vi "set_home_end.vi"(5 "End transform offset":dbl[](array[numeric])=[0.0, 0.0, 0.0, 0.0, 0.0, 0.0] format="%#.3f", 6 "End transform coordinates":T2(ring), 7 "Home pose offset":dbl[](array[numeric])=[0.0, 0.0, 0.0, 0.0, 0.0, 0.0] format="%#.3f", 9 "Probe pose (ASAP)":T1, 10 "Probe rotation (stage)":T1, 11 "Pivot point (mm)":dbl[](array[numeric])) -> (1 "End transform string":string, 2 "End transform":dbl[](array[numeric]), 3 "Home pose":dbl[](array[numeric]))   [LabVIEW 2013]
uses:
  <vilib>/Analysis/Matrix/Datatypes/RealMatrix.ctl
  <vilib>/Analysis/baseanly.llb/Real A x B.vi
  initialization/micron_globals.vi
  <vilib>/Analysis/NI_AALBase.lvlib
  <vilib>/Analysis/Matrix/NI_Matrix.lvlib
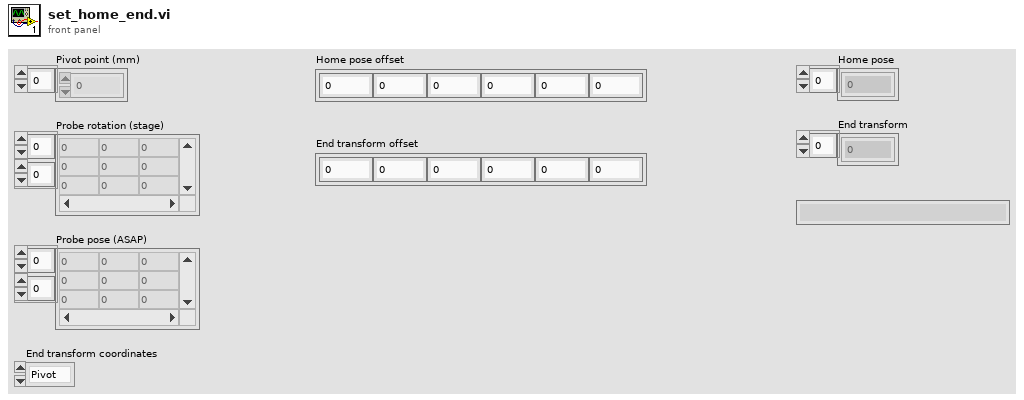
[diagram p1: front panel]
types:
  T1 = typedef "NI_Matrix.lvlib/RealMatrix.ctl" = dbl[][]
  T2 = enum16{"Pivot", "Probe", "ASAP", "Sensor 0", "Sensor 1"}
  T3 = typedef "configuration.ctl" = cluster{"Calibration data":T4, "Block size":i32, "Tasks":cluster{"Analog Input":refnum<k21>, "Counters":refnum<k21>[], "Digital out":refnum<k21>}, "Light enables":bool[]}
  T4 = typedef "asap_calibration.ctl" = cluster{"T1":T1, "K1":T1, "T2":T1, "K2":T1, "Sensor LUT":sgl[][][][]}
  T5 = typedef "motion_status.ctl" = cluster{"Axis names":string[], "Axis positions":dbl[], "Pose":dbl[], "Timestamp":u32, "Ready":bool, "Stopped":bool}
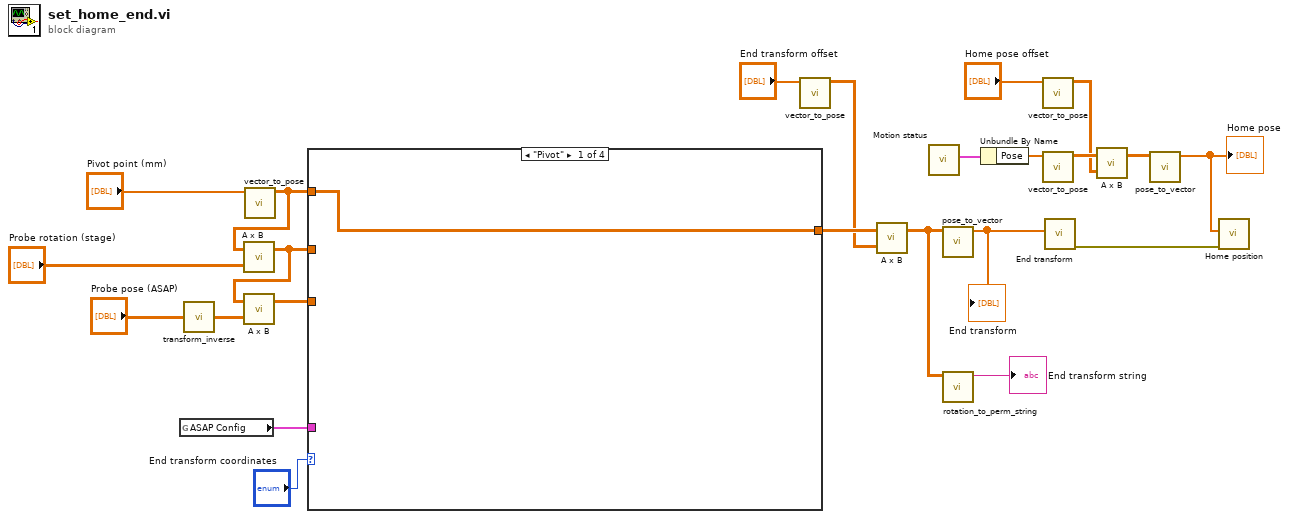
[diagram p0: block diagram]
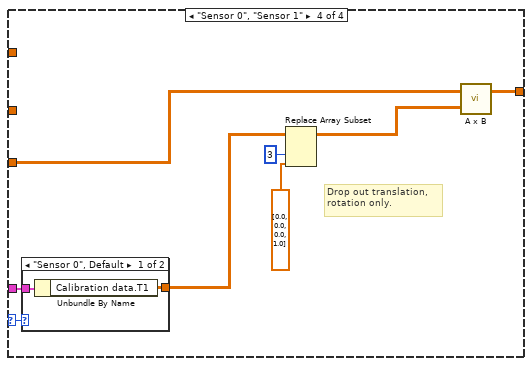
[diagram p4: hidden frame]
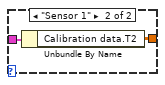
[diagram p5: hidden frame]
diagram:
  n1 = global read "micron_globals.vi" "ASAP Config"() -> (w13:T3)
  n2 = call "transform_inverse.vi"("Transform"="Probe pose (ASAP)") -> ("Inverse transform"=w21:T1)
  n3 = call "vector_to_pose.vi"("Pose vector"="Pivot point (mm)") -> ("Pose"=w19:T1)  [unwired: 10 in]
  n4 = call-poly <vilib>:"A x B.vi"("B"="Probe rotation (stage)", "A"=w19) -> ("A x B"=w22:T1)  [unwired: 1 out]
  n5 = call-poly <vilib>:"A x B.vi"("B"=w21, "A"=w22) -> ("A x B"=w23:T1)  [unwired: 1 out]
  n6 = case shown="\"Pivot\"" "End transform coordinates" {
    selector: "End transform coordinates" -> [_ _ _ w31]
    tunnel: w22 -> [_ w25 _ _]
    tunnel: [w24 w25 w26 w32] -> w10
    tunnel: w19 -> [w24 _ _ _]
    tunnel: w23 -> [_ _ w26 w33]
    tunnel: w13 -> [_ _ _ w34]
    frame "Pivot" {
    }
    frame "Probe" {
    }
    frame "ASAP" {
    }
    frame "Sensor 0", "Sensor 1" {
      # "Drop out translation, rotation only."
      n7 = case shown="\"Sensor 0\", Default" w31 {
        tunnel: w34 -> [w36 w38]
        tunnel: [w35 w37] -> w30
        frame "Sensor 0", Default {
          n8 = Unbundle By Name(w36) -> ("Calibration data.T1"=w35:T1)
        }
        frame "Sensor 1" {
          n9 = Unbundle By Name(w38) -> ("Calibration data.T2"=w37:T1)
        }
      }
      n10 = Replace Array Subset(array=w30, new element=dbl[] [0.0, 0.0, 0.0, 1.0] ("new element/subarray"), index (col)=3 ("disabled index (col)")) -> (w27:T1)  [unwired: 1 in]
      n11 = call-poly <vilib>:"A x B.vi"("B"=w27, "A"=w33) -> ("A x B"=w32:T1)  [unwired: 1 out]
    }
  }
  n12 = call "vector_to_pose.vi"("Pose vector"="End transform offset") -> ("Pose"=w8:T1)  [unwired: 10 in]
  n13 = call-poly <vilib>:"A x B.vi"("B"=w8, "A"=w10) -> ("A x B"=w7:T1)  [unwired: 1 out]
  n14 = call "Motion status.vi"() -> ("Motion status"=w14:T5)  [unwired: 6 in, 5 out]
  n15 = call "pose_to_vector.vi"("Pose"=w7) -> ("Pose vector"=w11:dbl[])  [unwired: 10 in]
  "End transform" <- w11
  n16 = call "rotation_to_perm_string.vi"("Rotation matrix (T)"=w7) -> ("Axis permutation and residue"=→"End transform string":string)  [unwired: 10 in]
  n17 = Unbundle By Name(w14) -> ("Pose"=w5:dbl[])
  n18 = call "vector_to_pose.vi"("Pose vector"="Home pose offset") -> ("Pose"=w3:T1)  [unwired: 10 in]
  n19 = call "vector_to_pose.vi"("Pose vector"=w5) -> ("Pose"=w4:T1)  [unwired: 10 in]
  n20 = call "End transform.vi"("End transform"=w11) -> ("error out"=w15:errorcluster)  [unwired: 10 in]
  n21 = call-poly <vilib>:"A x B.vi"("B"=w3, "A"=w4) -> ("A x B"=w2:T1)  [unwired: 1 out]
  n22 = call "pose_to_vector.vi"("Pose"=w2) -> ("Pose vector"=w1:dbl[])  [unwired: 10 in]
  "Home pose" <- w1
  n23 = call "Home position.vi"("error in"=w15, "Home position"=w1) -> ()  [unwired: 9 in, 1 out]
